vi "Multiply String.vi"(10 "y":string, 11 "x":string) -> (3 "x * y":string)   [LabVIEW 2013, in "Problem 20.lvlib"]
uses:
  Problem 20.lvlib
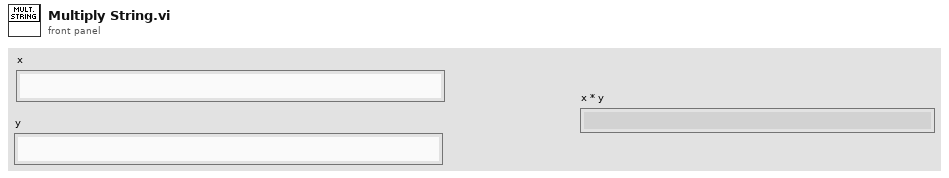
[diagram p1: front panel]
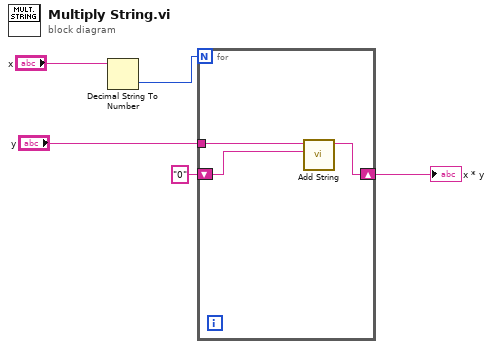
[diagram p0: block diagram]
diagram:
  n1 = Decimal String To Number(string="x") -> (number=w4:i32)  [unwired: 2 in, 1 out]
  n2 = for {
    N: w4 -> [_]
    tunnel: "y" -> [w8]
    shift-right: [w7] -> w2
    shift-left: "0" ("x + y") -> [w6]
    n3 = call "Add String.vi"("y"=w6, "x"=w8) -> ("x + y"=w7:string)  [unwired: 9 in]
  }
  "x * y" <- w2
